vi "FahrzustandSchaltungManuell.vi"(8 "Fahrzustand":T1, 10 "Geschwindigkeitsmultiplikator":dbl, 11 "Sensoren":dbl[](array[numeric])) -> (0 "PWM Motor":dbl, 1 "PWM Lenkung":dbl, 2 "Rundenzeiten":dbl[](array[numeric]), 3 "Linefollow_Array":bool[](array[boolean]))   [LabVIEW 2016]
uses:
  Control/Fahrart.ctl
  <vilib>/myRIO/Instrument Drivers/Onboard IO/DIO/typedefs/DIO Reference.ctl
  <vilib>/myRIO/Common/Instrument Driver Framework/Utilities/typedefs/myRIO Generic Hardware Reference.ctl
  <vilib>/myRIO/Common/Instrument Driver Framework/Utilities/typedefs/Hardware Version Enum.ctl
  <vilib>/myRIO/Common/Instrument Driver Framework/Utilities/typedefs/myRIO v1.0 Reference.ctl
  <vilib>/myRIO/Common/Instrument Driver Framework/Utilities/typedefs/Generic FPGA Reference.ctl
  <vilib>/myRIO/Common/Instrument Driver Framework/myRIO v1.0/DIO/typedefs/DIO Channels List.ctl
  <vilib>/myRIO/Common/Instrument Driver Framework/myRIO v1.0/DIO/typedefs/DIO Channels Enum.ctl
  <vilib>/userdefined/High Color/nirio_resource_hc.ctl
  <vilib>/myRIO/Common/Instrument Driver Framework/Utilities/vis/Is FPGA Ref Available.vi
  <vilib>/myRIO/Common/Instrument Driver Framework/myRIO v1.0/DIO/vis/myRIO v1.1 Open DIO.vi
  <vilib>/myRIO/Instrument Drivers/Onboard IO/DIO/vis/Write.vi
  <vilib>/myRIO/Common/Instrument Driver Framework/Utilities/vis/Validate Channels.vi
  <vilib>/myRIO/Common/Instrument Driver Framework/myRIO v1.0/DIO/vis/myRIO v1.0 Reserve DIO.vi
  <vilib>/myRIO/Common/Instrument Driver Framework/myRIO v1.0/Resource Manager/vis/myRIO v1.0 Reserve Channel List.vi
  <vilib>/myRIO/Common/Instrument Driver Framework/myRIO v1.0/DIO/vis/myRIO v1.0 Build MUX Configuration DIO.vi
  <vilib>/myRIO/Common/Instrument Driver Framework/myRIO v1.0/Resource Manager/vis/myRIO v1.0 Reserve Channel.vi
  <vilib>/myRIO/Common/Instrument Driver Framework/myRIO v1.0/Resource Manager/vis/myRIO v1.0 Unreserve Channel.vi
  <vilib>/myRIO/Common/Instrument Driver Framework/myRIO v1.0/Resource Manager/vis/myRIO v1.0 Create Configuration List.vi
  <vilib>/myRIO/Common/Instrument Driver Framework/myRIO v1.0/Resource Manager/vis/myRIO v1.0 Build Mutex Name.vi
  <vilib>/Utility/VariantDataType/GetNumericInfo.vi
  <vilib>/Utility/error.llb/Error Cluster From Error Code.vi
  <vilib>/myRIO/Common/Instrument Driver Framework/myRIO v1.0/myRIO v1.1 Open.vi
  <vilib>/myRIO/Common/Instrument Driver Framework/Utilities/vis/IO Manager.vi
  <vilib>/myRIO/Common/Instrument Driver Framework/Utilities/vis/Configuration Manager.vi
  <vilib>/myRIO/Common/Instrument Driver Framework/myRIO v1.0/Resource Manager/vis/myRIO v1.0 Configure IO.vi
  <vilib>/myRIO/Common/Instrument Driver Framework/myRIO v1.0/myRIO v1.0 Close.vi
  <vilib>/myRIO/Common/Instrument Driver Framework/myRIO v1.0/DIO/vis/myRIO v1.0 Write DIO.vi
  <vilib>/myRIO/Express VI/Onboard IO/DO/DO Express VI.xnode
  <vilib>/myRIO/Instrument Drivers/Onboard IO/DIO/vis/myRIO DIO Open.xnode
  <vilib>/myRIO/Instrument Drivers/Onboard IO/DIO/DIO.lvlib
panel:
  out "Position Strecke":dbl
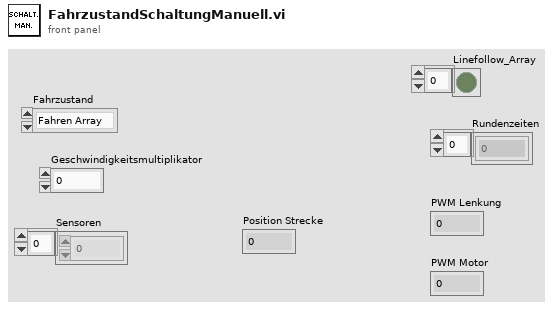
[diagram p1: front panel]
types:
  T1 = typedef "Fahrart.ctl" = enum16{"Fahren Array", "Folgen", "Überholen"}
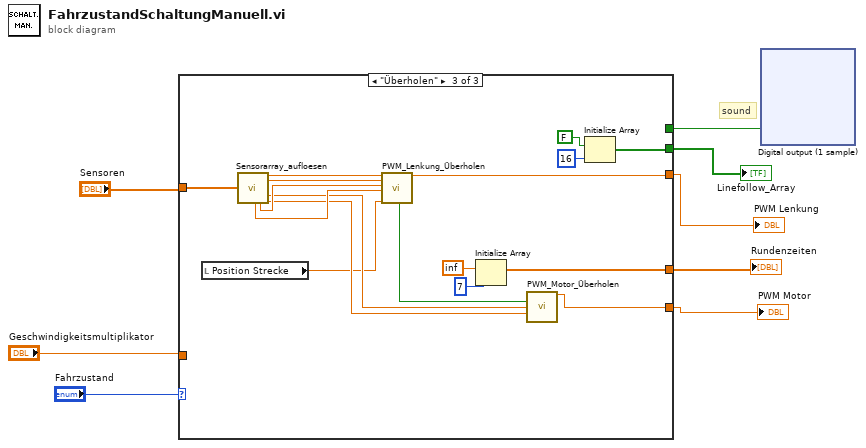
[diagram p0: block diagram]
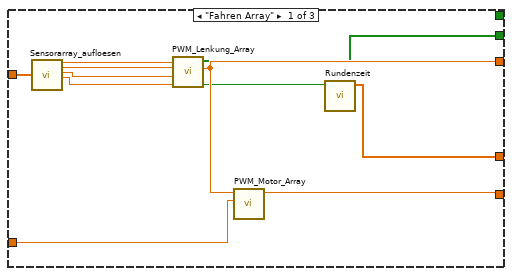
[diagram p2: hidden frame]
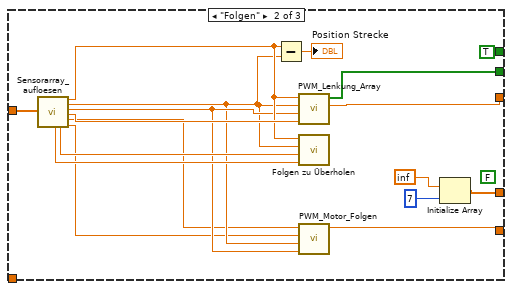
[diagram p3: hidden frame]
diagram:
  # "sound"
  n1 = case shown="\"Überholen\"" "Fahrzustand" {
    tunnel: "Geschwindigkeitsmultiplikator" -> [w18 _ _]
    tunnel: [w17 w36 w53] -> w1
    tunnel: [w19 w34 w52] -> w3
    tunnel: [w14 w32 w50] -> w2
    tunnel: [w16 w35 w49] -> w6
    tunnel: "Sensoren" -> [w9 w29 w45]
    tunnel: [_ TRUE _] -> w5
    frame "Fahren Array" {
      n2 = call "Sensorarray_aufloesen.vi"("Array"=w9) -> (14:w13:dbl, "vorne links"=w12:dbl, "schräg rechts"=w11:dbl, "schräg links"=w10:dbl)  [unwired: 11 in, 4 out]
      n3 = call "PWM_Lenkung_Array.vi"("schräg links"=w10, "schräg rechts"=w11, "vorne links"=w12, "vorne rechts"=w13) -> ("16 IR true"=w15:bool, "PWM Lenkung"=w19:dbl, "Linefollow_Array"=w16:bool[])  [unwired: 4 in]
      n4 = call "PWM_Motor_Array.vi"("Geschwindigkeit\nmultiplikator"=w18, "PWM Sensor"=w19) -> ("PWM Motor"=w17:dbl)  [unwired: 9 in]
      n5 = call "Rundenzeit.vi"("8 IR true"=w15) -> ("Rundenzeiten"=w14:dbl[])  [unwired: 10 in]
    }
    frame "Folgen" {
      (unwired) FALSE ("Back to Folgen")
      n6 = call "Sensorarray_aufloesen.vi"("Array"=w29) -> ("hinten links"=w25:dbl, "hinten rechts"=w26:dbl, 14:w27:dbl, "vorne links"=w23:dbl, "schräg rechts"=w24:dbl, "schräg links"=w28:dbl, "gerade rechts"=w22:dbl, "gerade links"=w21:dbl)  [unwired: 11 in]
      n7 = Subtract(x=w27, y=w23) -> (x-y=→"Position Strecke":dbl)
      n8 = call "PWM_Lenkung_Array.vi"("schräg links"=w28, "schräg rechts"=w24, "vorne links"=w23, "vorne rechts"=w27) -> ("PWM Lenkung"=w34:dbl, "Linefollow_Array"=w35:bool[])  [unwired: 4 in, 1 out]
      n9 = call "Folgen zu Überholen.vi"("hinten links"=w25, "hinten rechts"=w26, "vorne links"=w23, "vorne rechts"=w27) -> ()  [unwired: 7 in, 1 out]
      n10 = call "PWM_Motor_Folgen.vi"("Sensor gerade rechts"=w22, "Sensor gerade links"=w21, "Sensor schräg rechts"=w23, "Sensor schräg links"=w24) -> ("PWM Motor"=w36:dbl)  [unwired: 6 in]
      n11 = Initialize Array(inf, 7 ("dimension size")) -> (w32:dbl[])
    }
    frame "Überholen" {
      n12 = local read "Position Strecke"() -> (w37:dbl)
      n13 = call "Sensorarray_aufloesen.vi"("Array"=w45) -> ("hinten links"=w41:dbl, "hinten rechts"=w42:dbl, 14:w44:dbl, "vorne links"=w43:dbl, "gerade rechts"=w40:dbl, "gerade links"=w39:dbl)  [unwired: 11 in, 2 out]
      n14 = call "PWM_Lenkung_Überholen.vi"("vorne rechts"=w44, "vorne links"=w43, "hinten rechts"=w42, "hinten links"=w41, "Position Strecke"=w37) -> ("Abstand Bande erreicht"=w38:bool, "PWM Lenkung"=w52:dbl)  [unwired: 12 in, 1 out]
      n15 = Initialize Array(inf, 7 ("dimension size")) -> (w50:dbl[])
      n16 = call "PWM_Motor_Überholen.vi"("Boolean"=w38, "Sensor geradeaus rechts"=w40, "Sensor geradeaus links"=w39) -> ("PWM Motor"=w53:dbl)  [unwired: 12 in]
      n17 = Initialize Array(FALSE, 16 ("dimension size")) -> (w49:bool[])
    }
  }
  "Linefollow_Array" <- w6
  "Rundenzeiten" <- w2
  "PWM Motor" <- w1
  "PWM Lenkung" <- w3
  n18 = xnode "Digital output (1 sample)"("A/DIO9 (Pin 29)"=w5) -> ()  [unwired: 1 in, 1 out]
